vi "Shutdown.vi"(8 "error in (no error)":errorcluster, 9 "Message Data":variant, 10 "Name":string, 11 "Controller in":refnum<class "Controller.lvclass">) -> (0 "error out":errorcluster, 3 "Controller out":refnum<class "Controller.lvclass">)   [LabVIEW 2020, in "Controller.lvclass"]
uses:
  Controller.lvclass
  Controller.lvclass/Controller.ctl
  Module/Module.lvclass
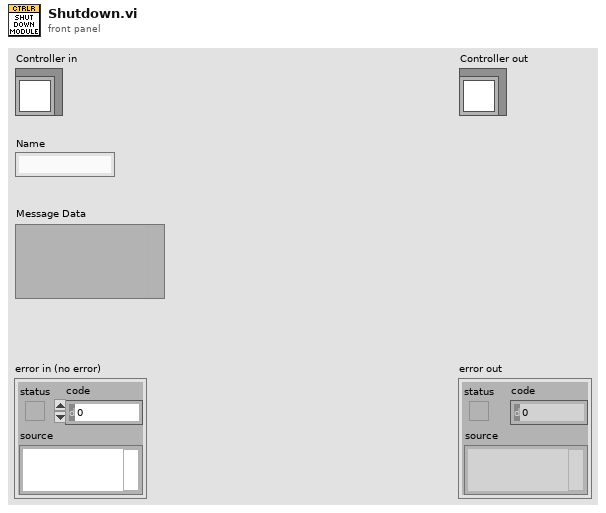
[diagram p1: front panel]
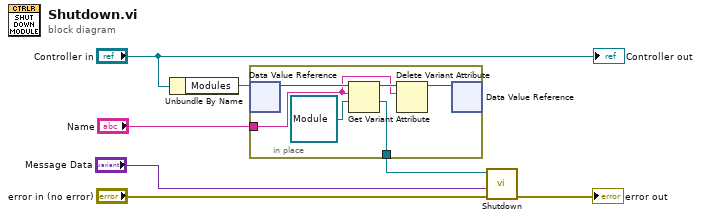
[diagram p0: block diagram]
diagram:
  n1 = Unbundle By Name("Controller in") -> ("Modules"=w2:refnum<data-value>)
  n2 = in-place {
    in-place-border: "Name" -> [w8]
    in-place-border: [w9] -> w1
    n3 = in-place-dvr #1(w2) -> (w12:variant)  [unwired: 1 out]
    n4 = Get Variant Attribute(Variant=w12, name=w8, default value (empty Variant)=refnum<class "Module.lvclass"> refnum ("Module.lvclass")) -> (duplicate Variant=w11:variant, value=w9:refnum<class "Module.lvclass">)  [unwired: 1 in, 2 out]
    n5 = Delete Variant Attribute(6:w8, 7:w11) -> (3:w13:variant)  [unwired: 1 in, 2 out]
    n6 = in-place-dvr #1(w13) -> ()  [unwired: 2 out]
  }
  n7 = call "Shutdown.vi"("error in (no error)"="error in (no error)", "Params"="Message Data", "Module in"=w1) -> ("error out"=→"error out":errorcluster)  [unwired: 7 in, 1 out]
  "Controller out" <- "Controller in"
